vi "WASh simulated database.vi"(7 "task":T2, 8 "error in (no error)":errorcluster, 10 "datatbase record":T1 {"Step duration" format="%#_5f"}, 11 "Wash step name":string) -> (0 "error out":errorcluster, 1 "locked?":bool, 3 "Step duration":i32)   [LabVIEW 2018]
doc: "Simulates configuration database. In subsequent phases of the project only this Vi shall be modified to handle communication with the configuration database.\n\n[Covers: SI1]\n[Covers: SD1]"
uses:
  type defs/WASH simulated database tasks.ctl
  type defs/WASH database record.ctl
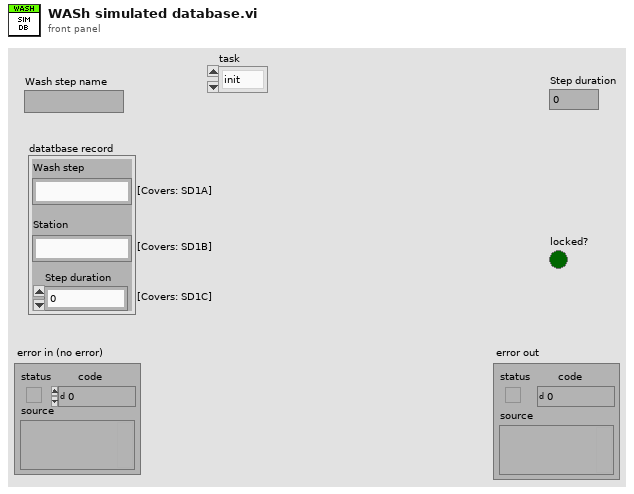
[diagram p1: front panel]
types:
  T1 = typedef "WASH database record.ctl" = cluster{"Wash step":string, "Station":string, "Step duration":i32}
  T2 = typedef "WASH simulated database tasks.ctl" = enum16{"init", "read", "insert record", "update record", "query timing", "close"}
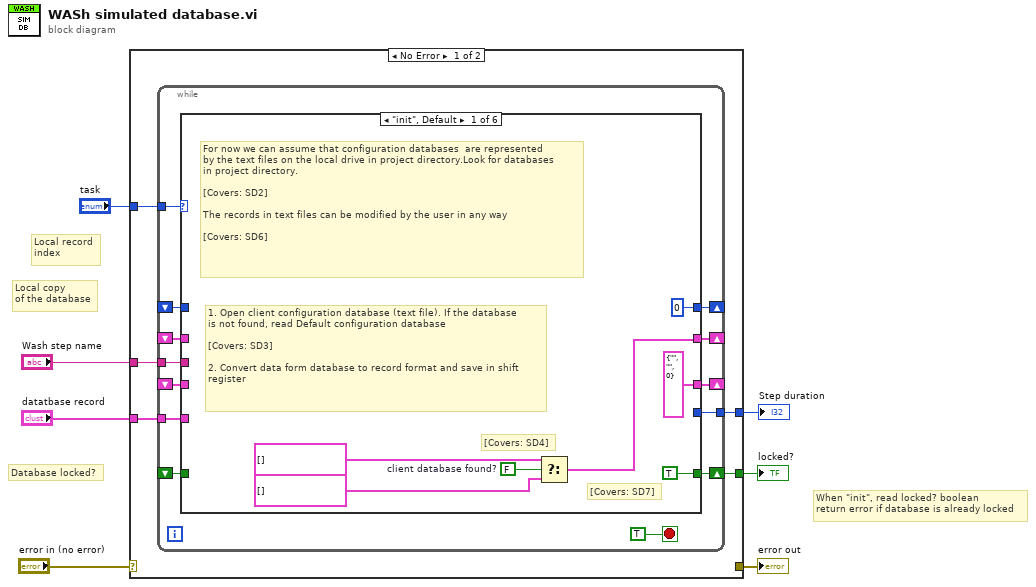
[diagram p0: block diagram]
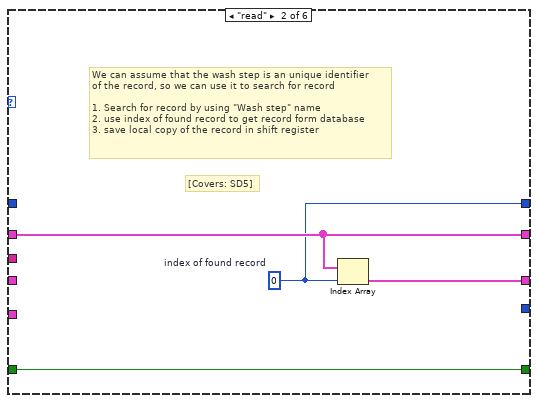
[diagram p2: hidden frame]
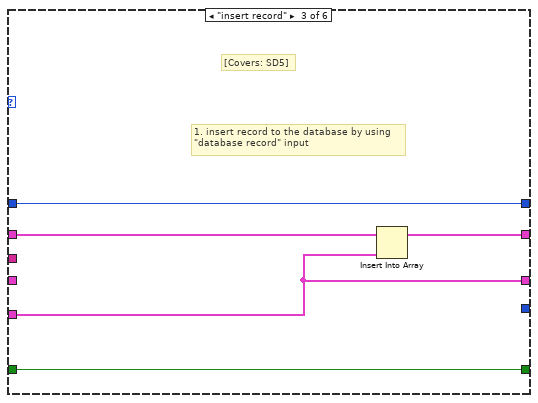
[diagram p3: hidden frame]
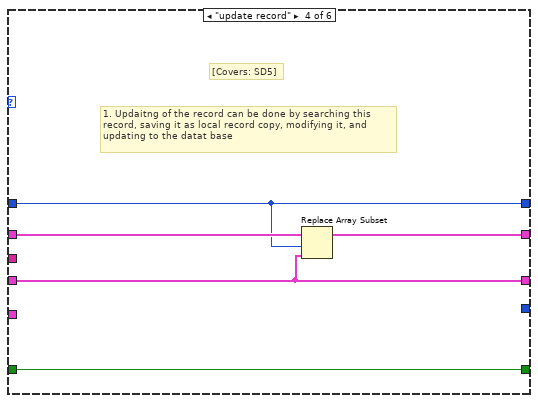
[diagram p4: hidden frame]
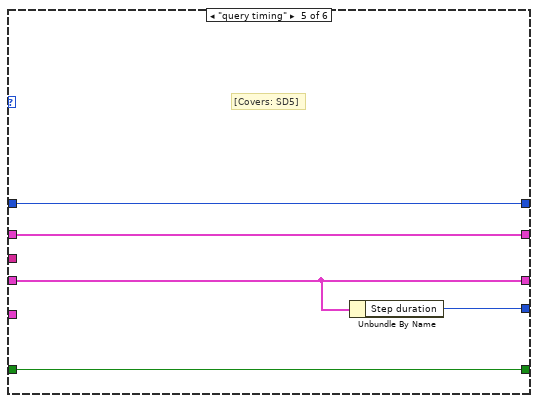
[diagram p5: hidden frame]
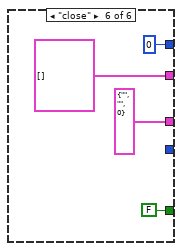
[diagram p6: hidden frame]
diagram:
  # "When \"init\", read locked? boolean\nreturn error if database is already locked"
  # "Local record\nindex"
  # "Local copy\nof the database"
  # "Database locked?"
  n1 = case shown="No Error" "error in (no error)" {
    selector: "error in (no error)" -> [_ w56]
    tunnel: [_ w56] -> w6
    tunnel: "task" -> [w12 _]
    tunnel: "Wash step name" -> [w11 _]
    tunnel: [w10 _] -> w3
    tunnel: [w9 _] -> w2
    tunnel: "datatbase record" -> [w8 _]
    frame No Error {
      n2 = while {
        tunnel: w12 -> [w24]
        shift-right: [w23] -> _
        shift-left: _ -> [w20]
        tunnel: w11 -> [w22]
        shift-right: [w21] -> w10
        shift-left: _ -> [w16]
        shift-right: [w19] -> _
        shift-left: _ -> [w18]
        tunnel: [w17] -> w9
        tunnel: w8 -> [w15]
        shift-right: [w14] -> _
        shift-left: _ -> [w13]
        stop <- TRUE stop-if-true
        n3 = case shown="\"init\", Default" w24 {
          tunnel: [w30 w36 w39 w43 w48 T1[] [] ("t")] -> w23
          tunnel: w22 -> [_ _ _ _ _ _]
          tunnel: [TRUE w33 w38 w42 w49 FALSE] -> w21
          tunnel: w20 -> [_ w36 w41 w46 w48 _]
          tunnel: [T1 {"Wash step"="", "Station"="", "Step duration"=0} ("datatbase record") w35 w40 w45 w51 T1 {"Wash step"="", "Station"="", "Step duration"=0} ("datatbase record")] -> w19
          tunnel: w18 -> [_ _ _ w45 w51 _]
          tunnel: [_ _ _ _ w50 _] -> w17
          tunnel: w16 -> [_ w33 w38 w42 w49 _]
          tunnel: w15 -> [_ _ w40 _ _ _]
          tunnel: [0 ("index of found record") w34 w37 w44 w47 0 ("index of found record")] -> w14
          tunnel: w13 -> [_ _ w37 w44 w47 _]
          frame "init", Default {
            w31 = FALSE  # client database found?
            # "[Covers: SD7]"
            # "[Covers: SD4]"
            # "For now we can assume that configuration databases  are represented\nby the text files on the local drive in project directory.Look for databases\nin project directory.\n\n[Covers: SD2]\n\nThe records in text files can be modified by the user in any way\n\n[Covers: SD6]"
            # "1. Open client configuration database (text file). If the database\nis not found, read Default configuration database\n\n[Covers: SD3]\n\n2. Convert data form database to record format and save in shift\nregister"
            n4 = Select(t=T1[] [], s=w31, f=T1[] [] ("t")) -> (s? t:f=w30:T1[])
          }
          frame "read" {
            w34 = 0  # index of found record
            # "[Covers: SD5]"
            # "We can assume that the wash step is an unique identifier\nof the record, so we can use it to search for record\n\n1. Search for record by using \"Wash step\" name\n2. use index of found record to get record form database\n3. save local copy of the record in shift register"
            n5 = Index Array(array=w36, index=w34) -> (element=w35:T1)
          }
          frame "insert record" {
            # "1. insert record to the database by using\n\"database record\" input"
            # "[Covers: SD5]"
            n6 = Insert Into Array(array=w41, new element=w40) -> (w39:T1[])  [unwired: 1 in]
          }
          frame "update record" {
            # "1. Updaitng of the record can be done by searching this\nrecord, saving it as local record copy, modifying it, and\nupdating to the datat base"
            # "[Covers: SD5]"
            n7 = Replace Array Subset(array=w46, new element=w45, index=w44) -> (w43:T1[])
          }
          frame "query timing" {
            # "[Covers: SD5]"
            n8 = Unbundle By Name(w51) -> ("Step duration"=w50:i32)
          }
          frame "close" {
          }
        }
      }
    }
    frame Error {
    }
  }
  "error out" <- w6
  "locked?" <- w3
  "Step duration" <- w2
